vi "camera_load.vi"(7 "error in (no error)":errorcluster, 10 "path":path) -> (0 "error out":errorcluster, 1 "serials":u64[](array[numeric]) format="%.0x", 2 "sdks":string[](array[string]), 3 "names":string[](array[string]), 4 "ports":string[](array[string]), 5 "zlock":string, 6 "hdf":path)   [LabVIEW 2010]
uses:
  <vilib>/addons/h5labview2/base/hid_t.ctl
  <vilib>/addons/h5labview2/dataset/H5Dread.llb/H5Dread.xnode
  <vilib>/addons/h5labview2/attrib/H5Aread.llb/H5Aread.xnode
  <vilib>/Utility/config.llb/Read Key (String).vi
  <vilib>/addons/h5labview2/base/lib_path.vi
  <vilib>/addons/h5labview2/base/H5Equery.vi
  <vilib>/Utility/config.llb/NI_LVConfig.lvlib
  <vilib>/addons/h5labview2/file/H5F.lvlib
  <vilib>/addons/h5labview2/group/H5G.lvlib
panel:
  out "name":string
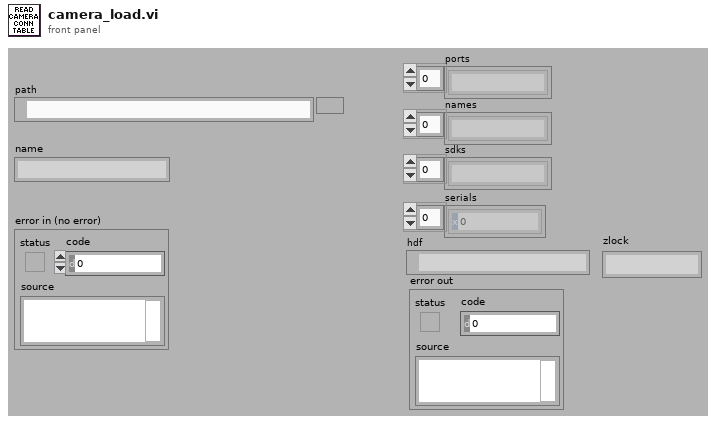
[diagram p1: front panel]
types:
  T1 = typedef "NI_LVConfig.lvlib/Config Data RefNum.ctl" = refnum<k1>
  T2 = typedef "hid_t.ctl" = i32
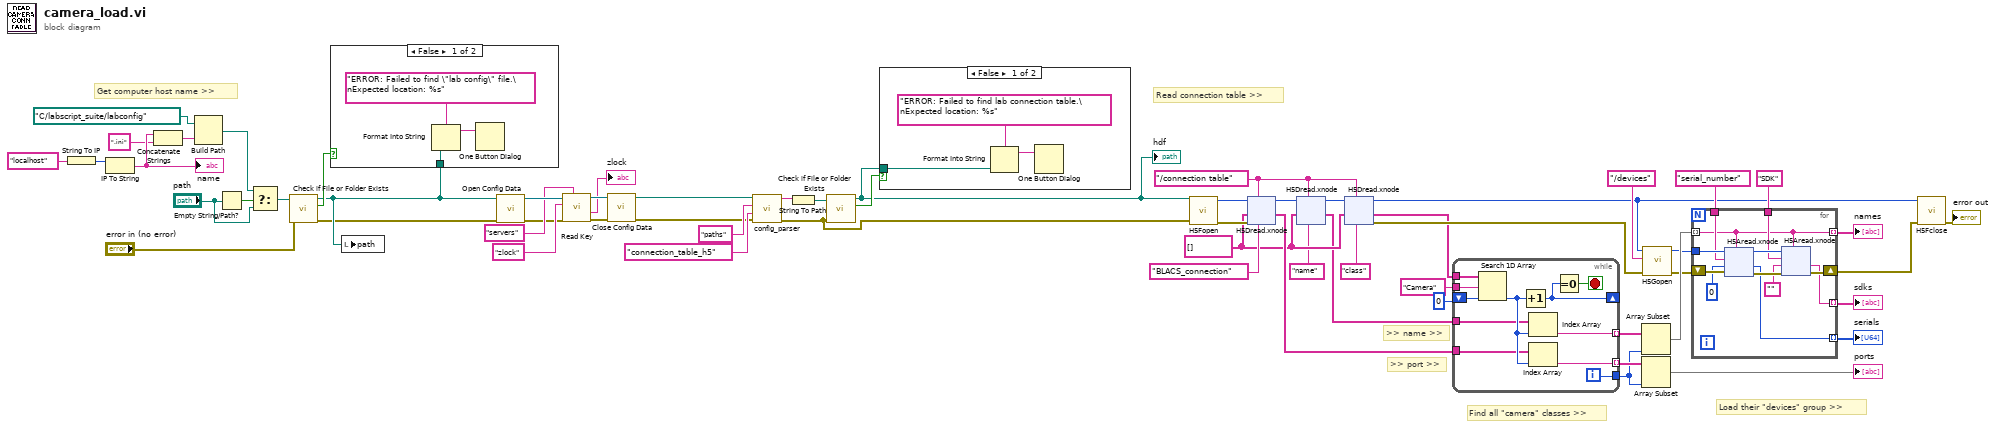
[diagram p0: block diagram]
diagram:
  w6 = string[] []
  w3 = "/connection table" ("table")
  # "Load their \"devices\" group >>"
  # "Find all \"camera\" classes >>"
  # "Read connection table >>"
  # "Get computer host name >>"
  # ">> name >>"
  # ">> port >>"
  n1 = String To IP(1:"localhost" ("name")) -> (0:w46:u32)
  n2 = IP To String(2:w46) -> (0:w44:string)  [unwired: 1 in]
  "name" <- w44
  n3 = Concatenate Strings(w44, ".ini" ("string")) -> (w42:string)
  n4 = Build Path(base path=path "C:/labscript_suite/labconfig", name or relative path=w42) -> (appended path=w40:path)
  n5 = Empty String/Path?(string/path="path") -> (empty?=w39:bool)
  n6 = Select(t=w40, s=w39, f="path") -> (s? t:f=w37:path)
  n7 = call <vilib>:"Check if File or Folder Exists.vi"("error in (no error)"="error in (no error)", "path"=w37) -> ("error out"=w23:errorcluster, "file or folder exists?"=w36:bool, "dup path"=w32:path)  [unwired: 7 in]
  n8 = case shown="False" w36 {
    tunnel: w32 -> [w63 _]
    frame False {
      n9 = Format Into String(format string="ERROR: Failed to find \"lab config\" file.\nExpected location: %s", w63) -> (resulting string=w62:string)  [unwired: 2 in, 1 out]
      n10 = One Button Dialog(message=w62) -> ()  [unwired: 1 in, 1 out]
    }
    frame True {
    }
  }
  n11 = local write "path"(w32) -> ()
  n12 = call <vilib>:"Open Config Data.vi"("error in (no error)"=w23, "configuration file path"=w32) -> ("error out"=w24:errorcluster, "refnum"=w31:T1)  [unwired: 7 in, 1 out]
  n13 = call-poly <vilib>:"Read Key.vi"("section"="servers", "error in (no error)"=w24, "key"="zlock", "refnum"=w31) -> ("error out"=w29:errorcluster, "value"=→"zlock":string, "refnum out"=w30:T1)  [unwired: 4 in, 1 out]
  n14 = call <vilib>:"Close Config Data.vi"("error in (no error)"=w29, "refnum"=w30) -> ("error out"=w27:errorcluster, "file path"=w28:path)  [unwired: 8 in]
  n15 = call <userlib>:"config_parser.vi"("error in"=w27, "key"="connection_table_h5", "section"="paths", "path"=w28) -> ("error out"=w21:errorcluster, "result"=w59:string)  [unwired: 2 in]
  n16 = String To Path(string=w59) -> (path=w35:path)
  n17 = call <vilib>:"Check if File or Folder Exists.vi"("error in (no error)"=w21, "path"=w35) -> ("file or folder exists?"=w34:bool, "dup path"=w20:path)  [unwired: 7 in, 1 out]
  "hdf" <- w20
  n18 = case shown="False" w34 {
    tunnel: w20 -> [w66 _]
    frame False {
      n19 = Format Into String(format string="ERROR: Failed to find lab connection table.\nExpected location: %s", w66) -> (resulting string=w65:string)  [unwired: 2 in, 1 out]
      n20 = One Button Dialog(message=w65) -> ()  [unwired: 1 in, 1 out]
    }
    frame True {
    }
  }
  n21 = call <vilib>:"H5Fopen.vi"("error in (no error)"=w21, "path"=w20) -> ("error out"=w12:errorcluster, "ref out"=w13:T2)  [unwired: 8 in]
  n22 = xnode "H5Dread.xnode"("type name (default)"="BLACS_connection", "dataset name (this)"=w3, "error in (no error)"=w12, "default"=w6, "ref in"=w13) -> ("data"=w7:string[], "ref out"=w9:T2)  [unwired: 1 in, 2 out]
  n23 = xnode "H5Dread.xnode"("type name (default)"="name", "dataset name (this)"=w3, "default"=w6, "ref in"=w9) -> ("data"=w5:string[], "ref out"=w8:T2)  [unwired: 2 in, 2 out]
  n24 = xnode "H5Dread.xnode"("type name (default)"="class", "dataset name (this)"=w3, "default"=w6, "ref in"=w8) -> ("error out"=w10:errorcluster, "data"=w4:string[], "ref out"=w11:T2)  [unwired: 2 in, 1 out]
  n25 = while {
    tunnel: w4 -> [w78]
    tunnel: "Camera" ("element") -> [w77]
    shift-right: [w74] -> _
    shift-left: 0 ("index of element") -> [w76]
    tunnel: w5 -> [w72]
    tunnel: w7 -> [w71]
    tunnel: [w70] -> w56 mode=indexing
    tunnel: [w69] -> w55 mode=indexing
    tunnel: [w68] -> w54
    i -> [w68]
    stop <- w75 stop-if-true
    n26 = Search 1D Array(1D array=w78, element=w77, start index (0)=w76) -> (index of element=w73:i32)
    n27 = Increment(x=w73) -> (x+1=w74:i32)
    n28 = Index Array(array=w72, index=w73) -> (element=w70:string)
    n29 = Index Array(array=w71, index=w73) -> (element=w69:string)
    n30 = Equal To 0?(x=w74) -> (x = 0?=w75:bool)
  }
  n31 = Array Subset(array=w56, length=w54) -> (w53:string[])  [unwired: 1 in]
  n32 = Array Subset(array=w55, length=w54) -> (→"ports":string[])  [unwired: 1 in]
  n33 = call <vilib>:"H5Gopen.vi"("error in (no error)"=w10, "name"="/devices", "ref in"=w11) -> ("error out"=w15:errorcluster, "group out"=w16:T2)  [unwired: 7 in]
  n34 = for {
    tunnel: w16 -> [w90]
    tunnel: w53 -> [w79] mode=indexing
    tunnel: "serial_number" ("attrib_name") -> [w88]
    tunnel: "SDK" ("attrib_name") -> [w85]
    tunnel: [w79] -> w49 mode=indexing
    tunnel: [w81] -> w48 mode=indexing
    tunnel: [w83] -> w47 mode=indexing
    shift-right: [w82] -> w18
    shift-left: w15 -> [w89]
    n35 = xnode "H5Aread.xnode"("object name"=w79, "error in (no error)"=w89, "default"=u64 0, "attrib name"=w88, "ref in"=w90) -> ("error out"=w87:errorcluster, "data"=w83:u64, "ref out"=w86:T2)  [unwired: 1 in, 1 out]
    n36 = xnode "H5Aread.xnode"("object name"=w79, "error in (no error)"=w87, "default"="", "attrib name"=w85, "ref in"=w86) -> ("error out"=w82:errorcluster, "data"=w81:string)  [unwired: 1 in, 2 out]
  }
  "names" <- w49
  "sdks" <- w48
  "serials" <- w47
  n37 = call <vilib>:"H5Fclose.vi"("error in (no error)"=w18, "ref"=w11) -> ("error out"=→"error out":errorcluster)  [unwired: 9 in]
